vi "Parse URL.vi"(8 "error in (no error)":errorcluster, 11 "WebSocket URL":string) -> (0 "error out":errorcluster, 1 "URI":string, 2 "host":string, 3 "protocol":string, 4 "port":u16)   [LabVIEW 2021, in "WebSockets.lvlib" / "WebSocket Client.lvclass"]
doc: "Parses the WebSockets URL to protocol (e.g. ws://), hostname, port and URI.\n\nPort defaults to 80 for ws:// and http:// and 443 for wss:// and https://\nWebSockets 2.0.1.40\nSam Sharp - MediaMongrels Ltd\nCopyright (c) 2019, MediaMongrels Ltd"
uses:
  WebSocket Client.lvclass
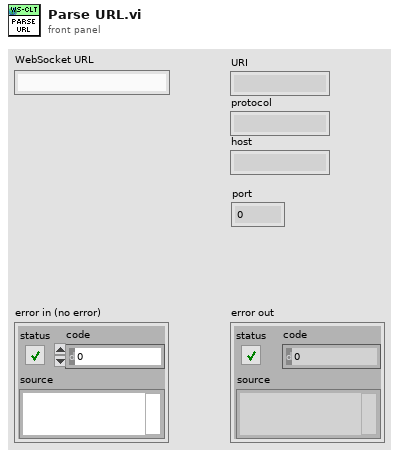
[diagram p1: front panel]
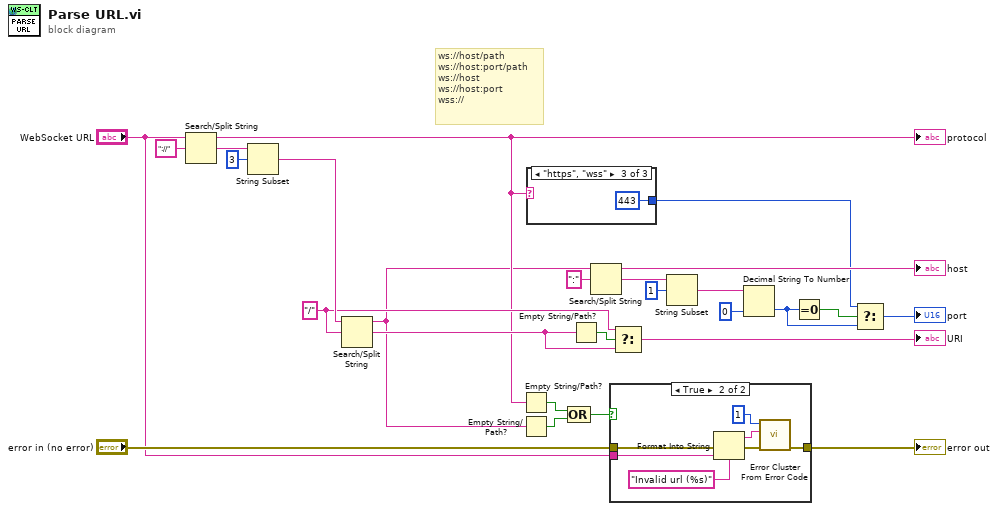
[diagram p0: block diagram]
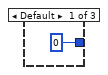
[diagram p2: hidden frame]
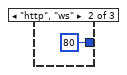
[diagram p3: hidden frame]
diagram:
  w14 = "/" ("search string/char (-)")
  # "ws://host/path\nws://host:port/path\nws://host\nws://host:port\nwss://"
  n1 = Search/Split String(string="WebSocket URL", search string/char (-)="://") -> (substring before match=w12:string, match + rest of string=w23:string)  [unwired: 1 in, 1 out]
  "protocol" <- w12
  n2 = String Subset(string=w23, offset (0)=3) -> (substring=w22:string)  [unwired: 1 in]
  n3 = Search/Split String(string=w22, search string/char (-)=w14) -> (substring before match=w11:string, match + rest of string=w15:string)  [unwired: 1 in, 1 out]
  n4 = Empty String/Path?(string/path=w12) -> (empty?=w21:bool)
  n5 = Empty String/Path?(string/path=w11) -> (empty?=w20:bool)
  n6 = case shown="\"https\", \"wss\"" w12 {
    tunnel: [u16 0 u16 80 u16 443] -> w4
    frame Default {
    }
    frame "http", "ws" {
    }
    frame "https", "wss" {
    }
  }
  n7 = Compound Arithmetic op=OR(w21, w20) -> (w17:bool)
  n8 = Empty String/Path?(string/path=w15) -> (empty?=w16:bool)
  n9 = Search/Split String(string=w11, search string/char (-)=":") -> (substring before match=→"host":string, match + rest of string=w8:string)  [unwired: 1 in, 1 out]
  n10 = case shown="True" w17 {
    tunnel: "error in (no error)" -> [w30 w37]
    tunnel: [w30 w36] -> w19
    tunnel: "WebSocket URL" -> [_ w33]
    frame False {
    }
    frame True {
      n11 = Format Into String(format string="Invalid url (%s)", error in=w37, w33) -> (resulting string=w34:string, error out=w35:errorcluster)  [unwired: 1 in]
      n12 = call <vilib>:"Error Cluster From Error Code.vi"("error in (no error)"=w35, "error message (\"\")"=w34, "error code (0)"=1) -> ("error out"=w36:errorcluster)  [unwired: 6 in]
    }
  }
  "error out" <- w19
  n13 = Select(t=w14, s=w16, f=w15) -> (s? t:f=→"URI":string)
  n14 = String Subset(string=w8, offset (0)=1) -> (substring=w6:string)  [unwired: 1 in]
  n15 = Decimal String To Number(string=w6, default (0L)=u16 0 ("default (0 I32)")) -> (number=w3:u16)  [unwired: 1 in, 1 out]
  n16 = Equal To 0?(x=w3) -> (x = 0?=w5:bool)
  n17 = Select(t=w4, s=w5, f=w3) -> (s? t:f=→"port":u16)
